vi "Dashboard.vi"() -> ()   [LabVIEW 2016, in "User Interface.lvlib"]
uses:
  User Interface.lvlib
  VI Name.ctl
  <vilib>/Utility/miscctls.llb/LVPointTypeDef.ctl
panel:
  out "Stop":bool
  in  "Recipe":bool
  in  "Report":bool
  in  "Maintenance":bool
  in  "Exit":bool
  in  "Inst Calibration":bool
  in  "Main_Test":bool
  in  "App Run Mode":enum16{"Simulation", "Hardware"}(ring)=enum."Hardware"
  out "Top Label":string="DASHBOARD"
  out "Time":string="Sat  8/3/2019  8:10:44 PM"
  out "error out":errorcluster
  in  "error in (no error)":errorcluster
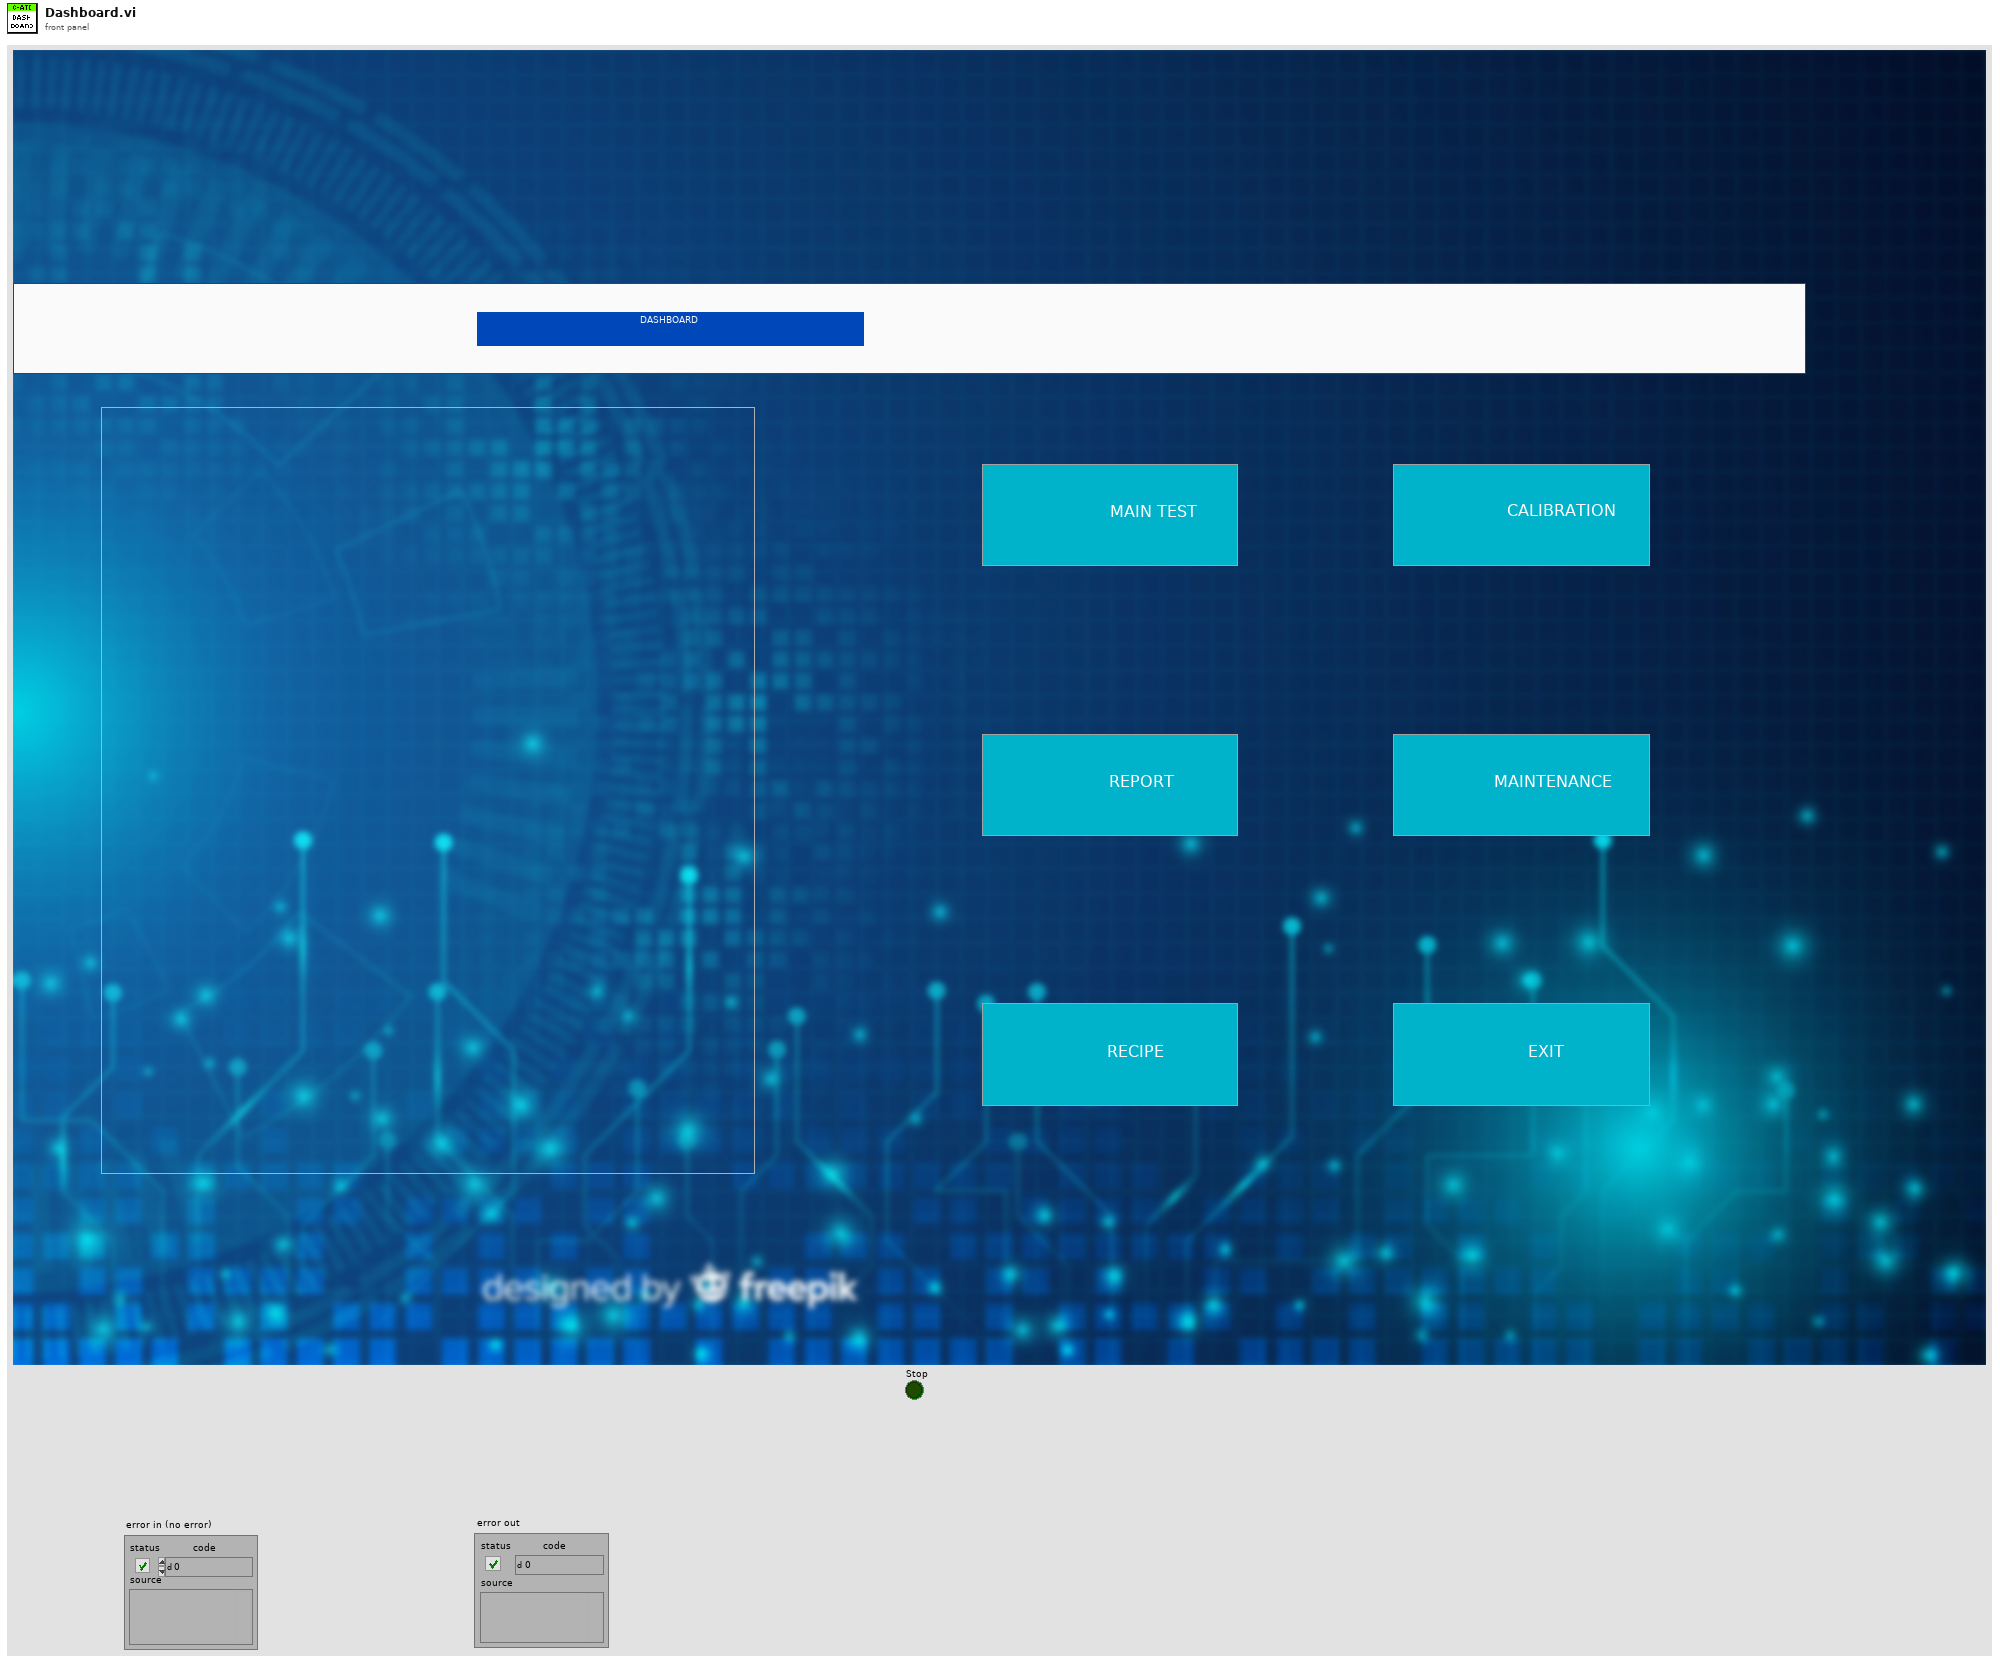
[diagram p1: front panel]
types:
  T1 = typedef "LVPointTypeDef.ctl" = cluster{"Horizontal":i16, "Vertical":i16}
  T2 = typedef "User Interface.lvlib/VI Name.ctl" = enum16{"Dashboard", "Maintenance", "Recipe", "Inst Calibration", "Testing", "Report"}
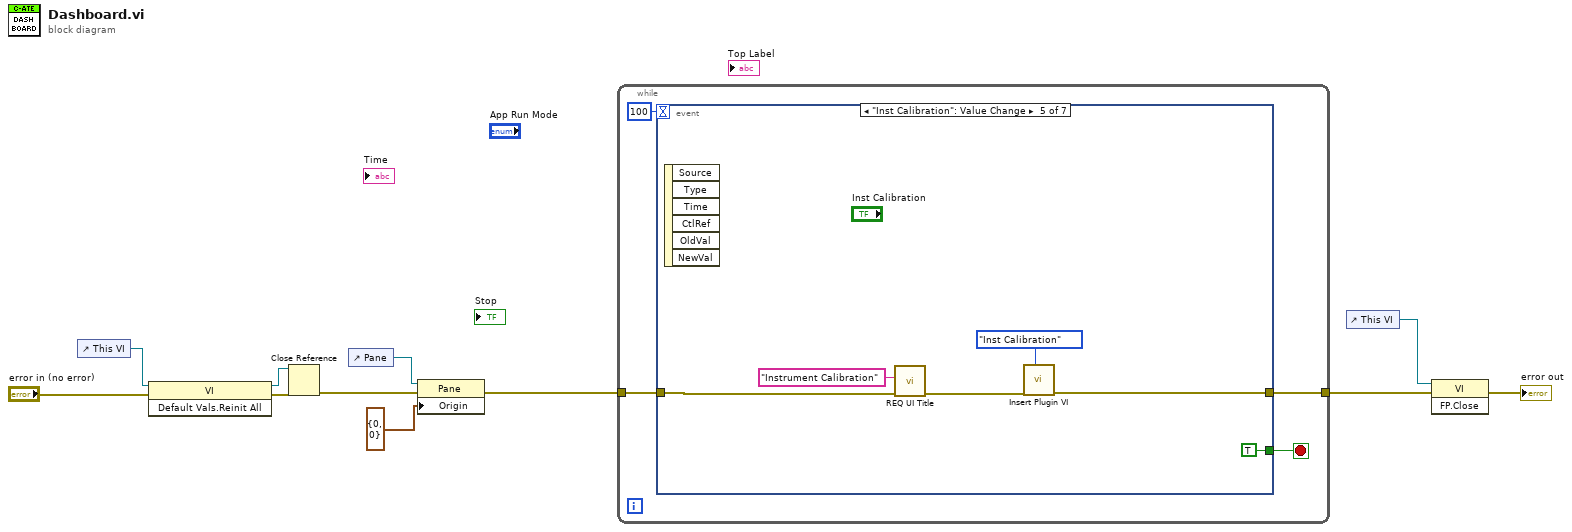
[diagram p0: block diagram]
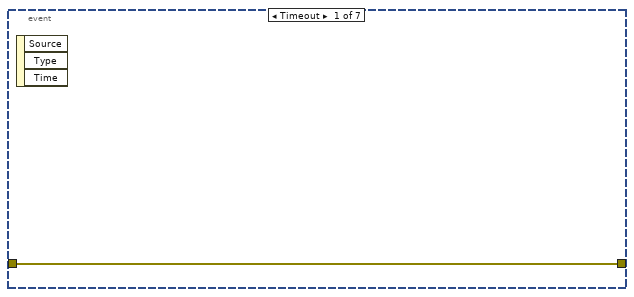
[diagram p2: hidden frame]
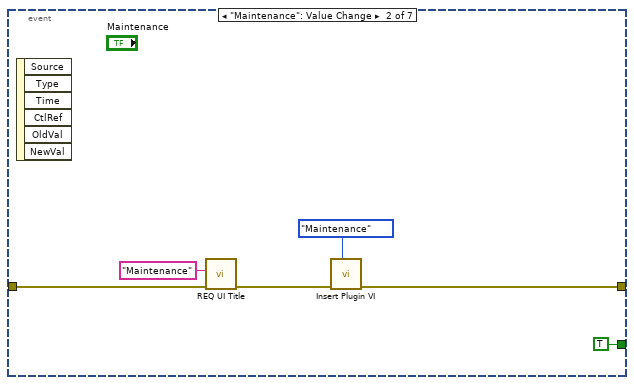
[diagram p3: hidden frame]
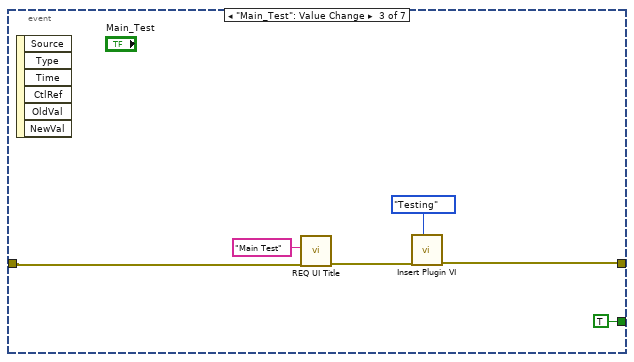
[diagram p4: hidden frame]
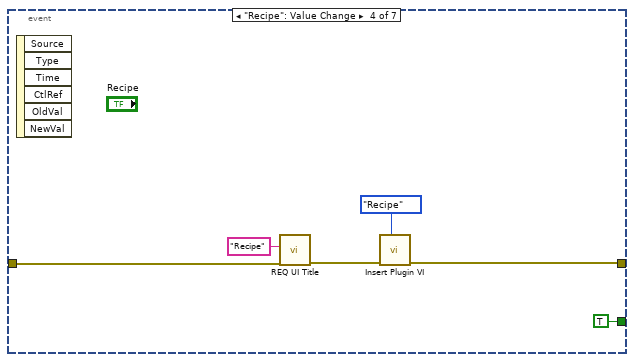
[diagram p5: hidden frame]
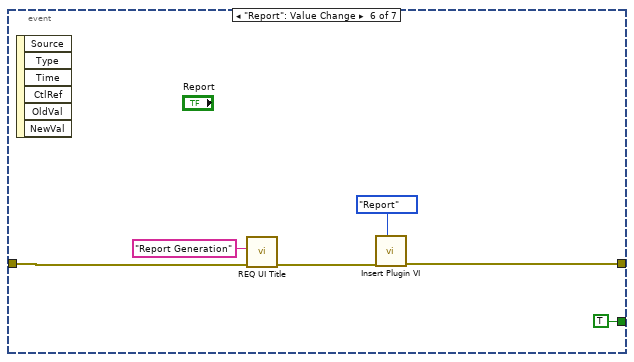
[diagram p6: hidden frame]
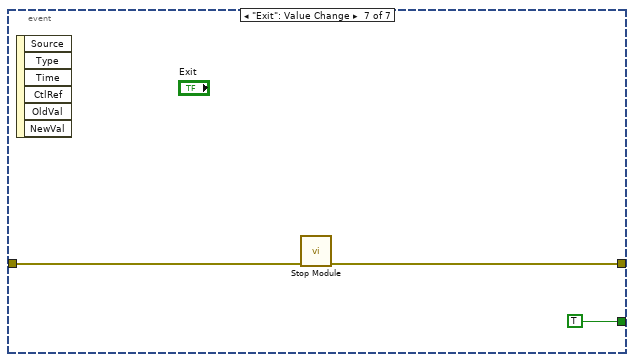
[diagram p7: hidden frame]
diagram:
  n1 = control-ref of="This VI"() -> (w5:refnum<vi>)
  n2 = invoke class="VI" method="Default Vals.Reinit All"(reference=w5, error in="error in (no error)") -> (reference out=w3:refnum<vi>, error out=w4:errorcluster)  [unwired: 1 in, 1 out]
  n3 = Close Reference(reference=w3, error in (no error)=w4) -> (error out=w1:errorcluster)
  n4 = control-ref of="Pane"() -> (w10:refnum<vi>)
  n5 = property class="Pane"(reference=w10, error in=w1, "Origin"=T1 {"Horizontal"=0, "Vertical"=0}) -> (error out=w11:errorcluster)  [unwired: 1 out]
  n6 = while {
    tunnel: w11 -> [w15]
    tunnel: [w13] -> w8
    stop <- w12 stop-if-true
    n7 = event shown="[4] \"Inst Calibration\": Value Change" {
      selector: _ -> [_ _ _ _ _ _ _]
      dyn-events: _ -> [_ _ _ _ _ _ _]
      timeout: 100 -> [_ _ _ _ _ _ _]
      tunnel: w15 -> [w16 w19 w24 w30 w37 w42 w48]
      tunnel: [w16 w21 w27 w33 w40 w45 w47] -> w13
      tunnel: [_ TRUE TRUE TRUE TRUE TRUE TRUE] -> w12
      event Timeout {
        n8 = event-data() -> ()  [unwired: 1 in, 3 out]
      }
      event "Maintenance": Value Change {
        n9 = event-data() -> ()  [unwired: 1 in, 6 out]
        n10 = call "REQ UI Title.vi"("error in"=w19, "UI Title"="Maintenance") -> ("error out"=w18:errorcluster)  [unwired: 9 in]
        n11 = call "Insert Plugin VI.vi"("VI Name"=VI_Name."Maintenance", "error in (no error)"=w18) -> ("error out"=w21:errorcluster)  [unwired: 9 in]
      }
      event "Main_Test": Value Change {
        n12 = event-data() -> ()  [unwired: 1 in, 6 out]
        n13 = call "REQ UI Title.vi"("error in"=w24, "UI Title"="Main Test") -> ("error out"=w23:errorcluster)  [unwired: 9 in]
        n14 = call "Insert Plugin VI.vi"("VI Name"=VI_Name."Testing", "error in (no error)"=w23) -> ("error out"=w27:errorcluster)  [unwired: 9 in]
      }
      event "Recipe": Value Change {
        n15 = event-data() -> ()  [unwired: 1 in, 6 out]
        n16 = call "REQ UI Title.vi"("error in"=w30, "UI Title"="Recipe") -> ("error out"=w29:errorcluster)  [unwired: 9 in]
        n17 = call "Insert Plugin VI.vi"("VI Name"=VI_Name."Recipe", "error in (no error)"=w29) -> ("error out"=w33:errorcluster)  [unwired: 9 in]
      }
      event "Inst Calibration": Value Change {
        n18 = event-data() -> ()  [unwired: 1 in, 6 out]
        n19 = call "REQ UI Title.vi"("error in"=w37, "UI Title"="Instrument Calibration") -> ("error out"=w36:errorcluster)  [unwired: 9 in]
        n20 = call "Insert Plugin VI.vi"("VI Name"=VI_Name."Inst Calibration", "error in (no error)"=w36) -> ("error out"=w40:errorcluster)  [unwired: 9 in]
      }
      event "Report": Value Change {
        n21 = event-data() -> ()  [unwired: 1 in, 6 out]
        n22 = call "REQ UI Title.vi"("error in"=w42, "UI Title"="Report Generation") -> ("error out"=w41:errorcluster)  [unwired: 9 in]
        n23 = call "Insert Plugin VI.vi"("VI Name"=VI_Name."Report", "error in (no error)"=w41) -> ("error out"=w45:errorcluster)  [unwired: 9 in]
      }
      event "Exit": Value Change {
        n24 = event-data() -> ()  [unwired: 1 in, 6 out]
        n25 = call "Stop Module.vi"("error in"=w48) -> ("error out"=w47:errorcluster)  [unwired: 10 in]
      }
    }
  }
  n26 = control-ref of="This VI"() -> (w6:refnum<vi>)
  n27 = invoke class="VI" method="FP.Close"(reference=w6, error in=w8) -> (error out=→"error out":errorcluster)  [unwired: 1 in, 2 out]
